vi "FPGA DAC IO Node.vi"(0 "data":T1[](array[typedef])=[{"I"=0.0, "Q"=0.0, "overflow"=FALSE}, {"I"=0.0, "Q"=0.0, "overflow"=FALSE}], 9 "input valid":bool, 11 "niUSRP Tx Core v1 FPGA.lvclass":refnum<class "niUSRP Tx Core v1 FPGA.lvclass">) -> ()   [LabVIEW 2025, in "niUSRP Tx Core v1 FPGA.lvclass"]
uses:
  niUSRP Tx Core v1 FPGA.lvclass
  <instrlib>/_niInstr/DSP/v1/Shared/Public/IQ Data.ctl
  <vilib>/rvi/eio/common/nirviEmuTemplateMethod_errors.vi
  <vilib>/eio/EIONode/EIONode.xnode
  <instrlib>/_niInstr/Basic Elements/v1/FPGA/niInstr Basic Elements v1 FPGA.lvlib
  <instrlib>/_niInstr/DSP/v1/Shared/niInstr DSP v1 Shared.lvlib
  <vilib>/rvi/DataTransferAndStorage/Container/XNode/niFpgaContainer.xnode
  <instrlib>/_niInstr/DSP/v1/FPGA/niInstr DSP v1 FPGA.lvlib
  <vilib>/rvi/FIFO/Fifo_Resource/niFpgaFifoEmulationRefIn.vi
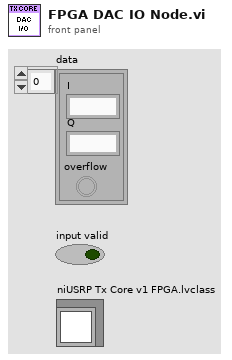
[diagram p1: front panel]
types:
  T1 = typedef "niInstr DSP v1 Shared.lvlib/IQ Data.ctl" = cluster{"I":fxp<+/-,18,1>, "Q":fxp<+/-,18,1>, "overflow":bool}
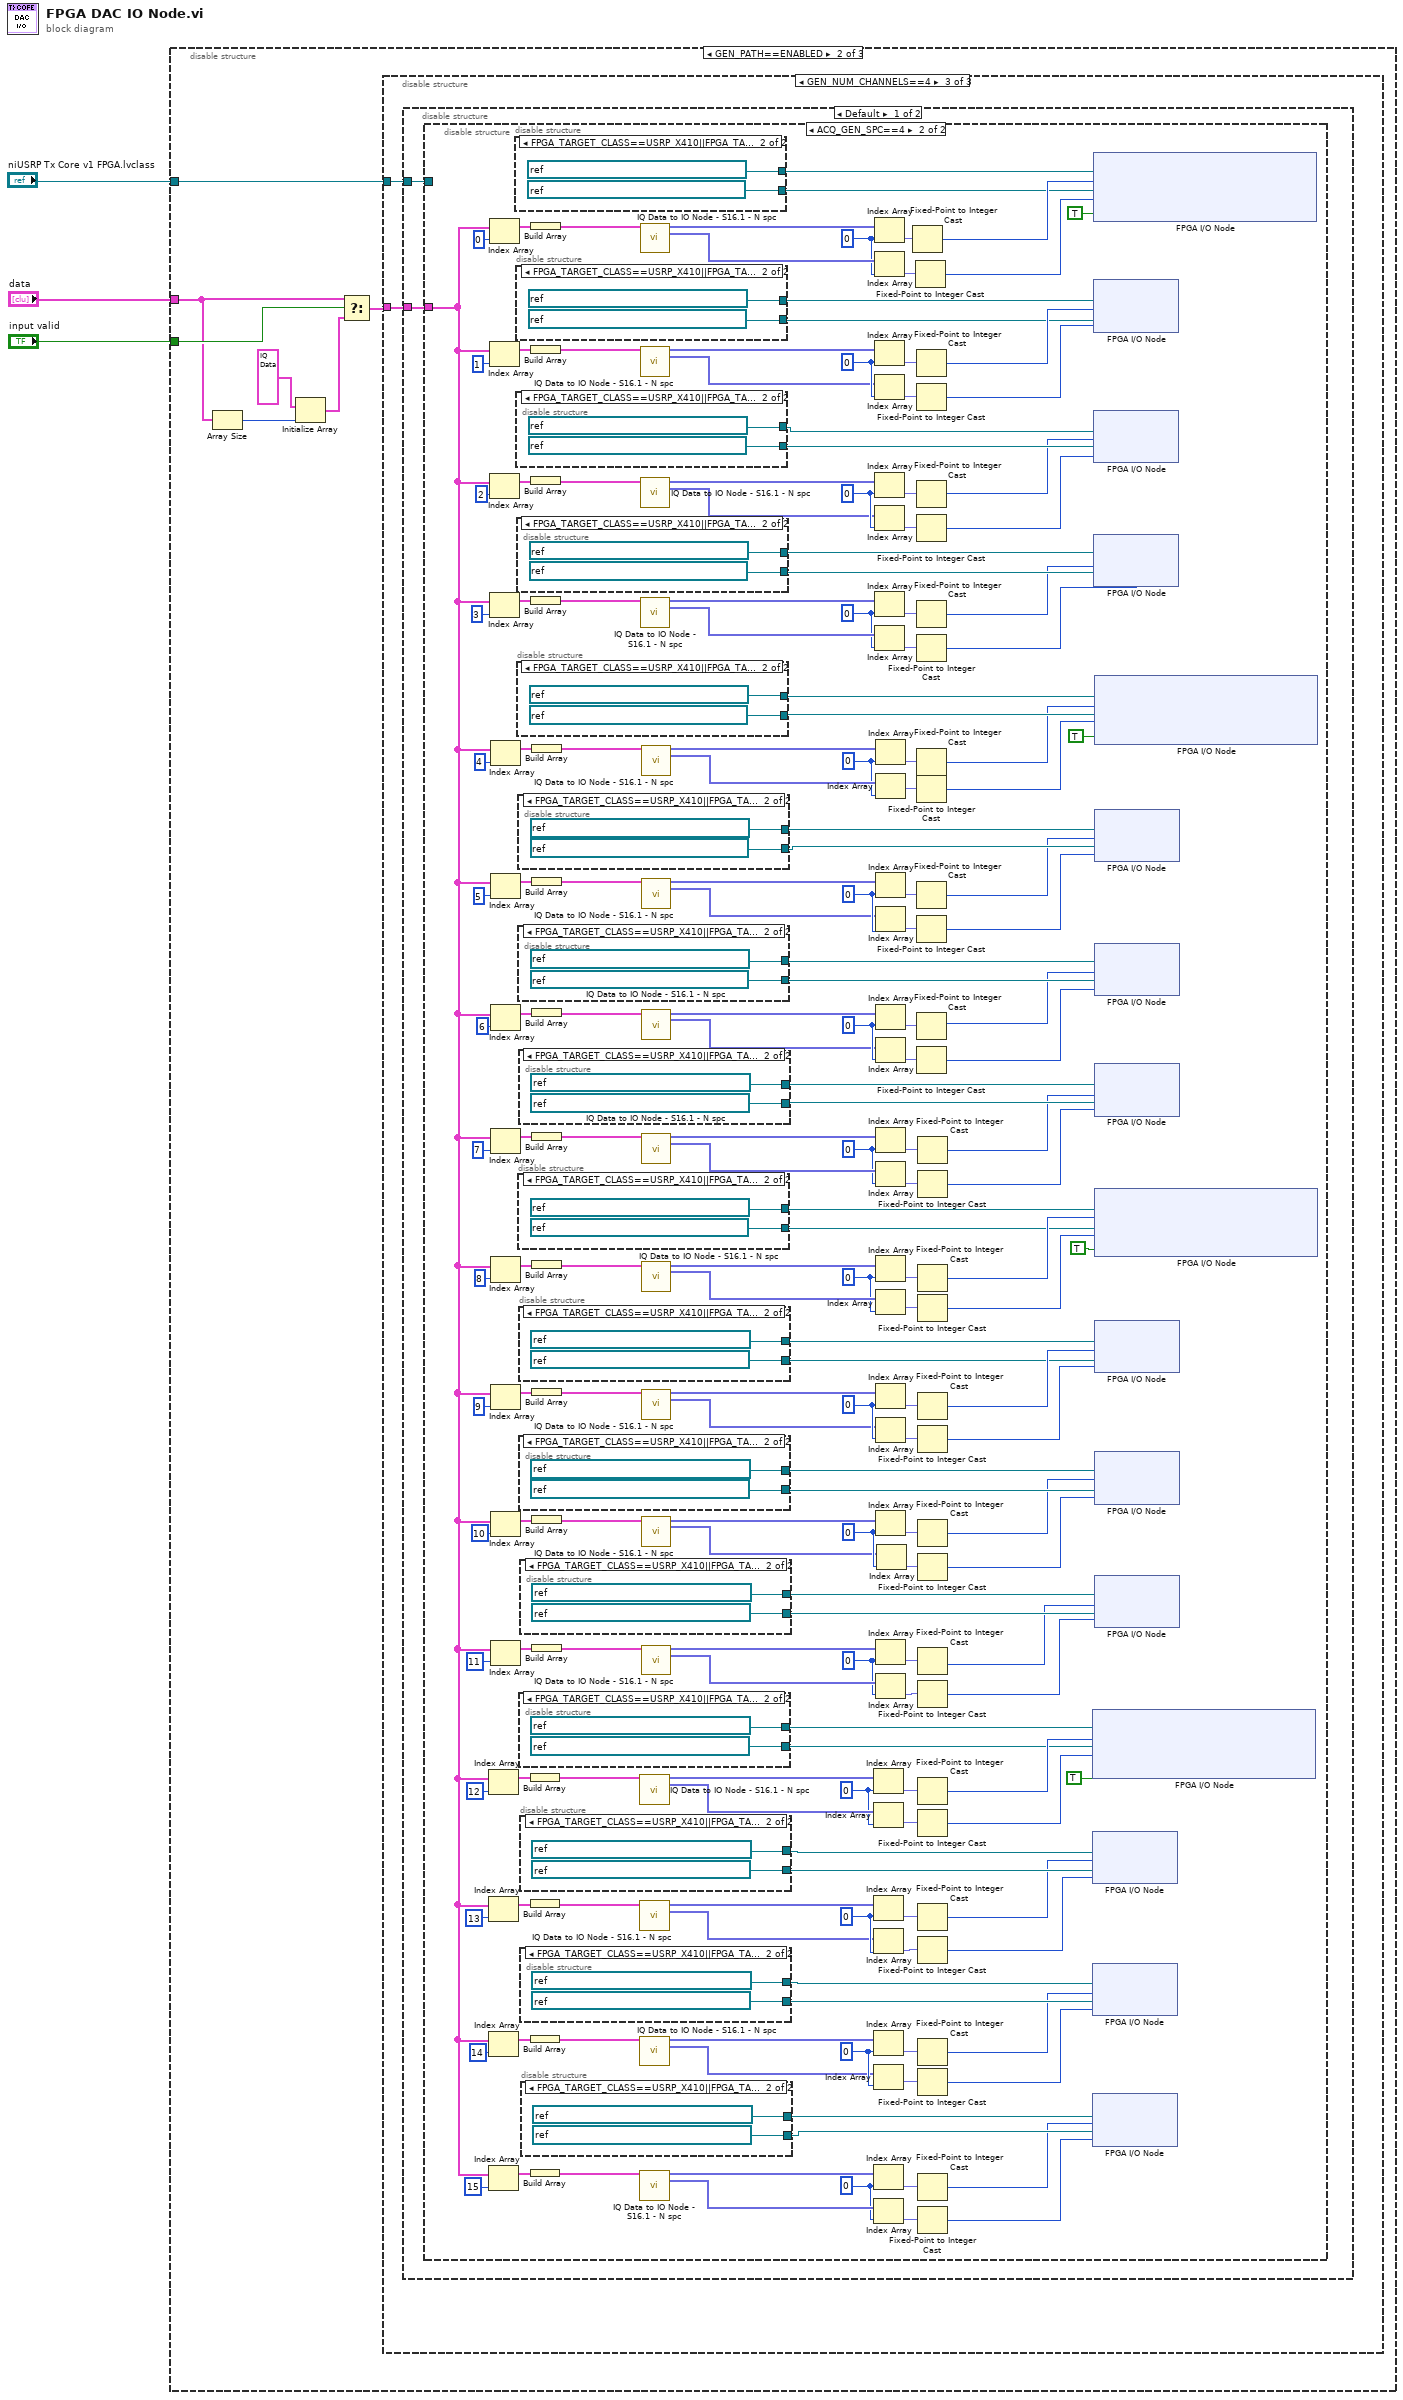
[diagram p0: block diagram]
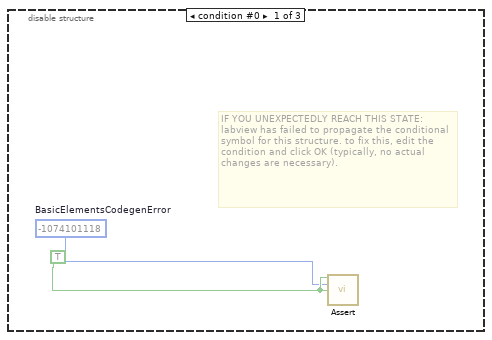
[diagram p2: hidden frame]
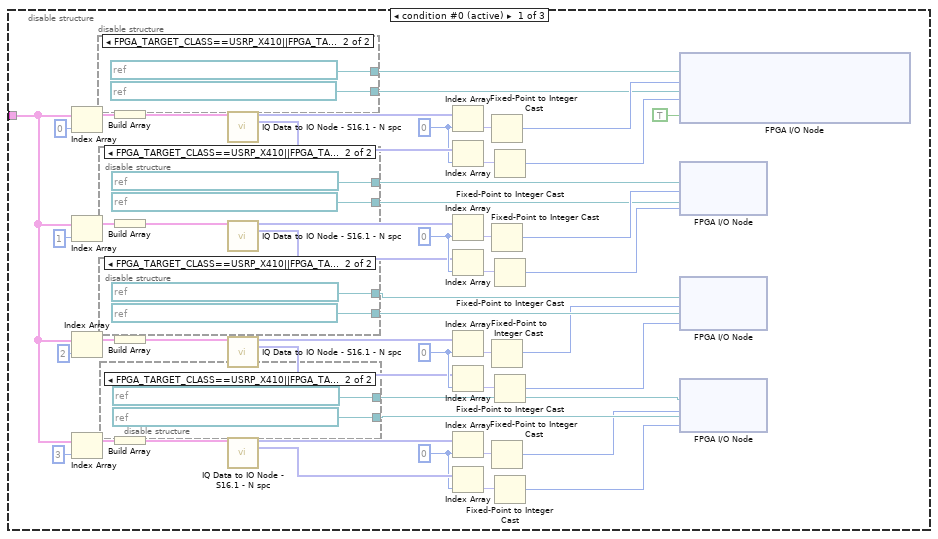
[diagram p4: hidden frame]
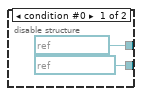
[diagram p5: hidden frame]
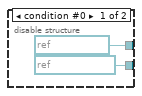
[diagram p6: hidden frame]
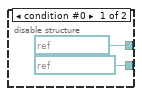
[diagram p7: hidden frame]
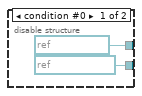
[diagram p8: hidden frame]
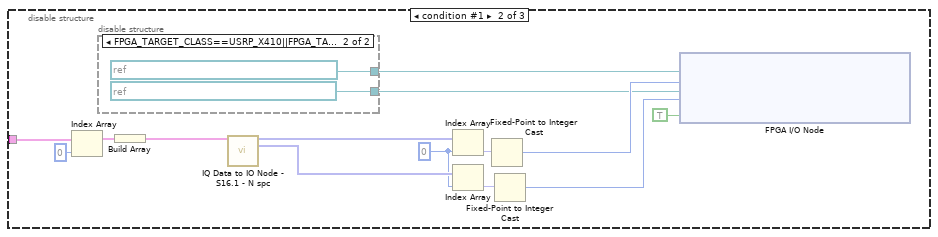
[diagram p9: hidden frame]
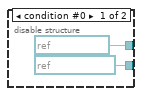
[diagram p10: hidden frame]
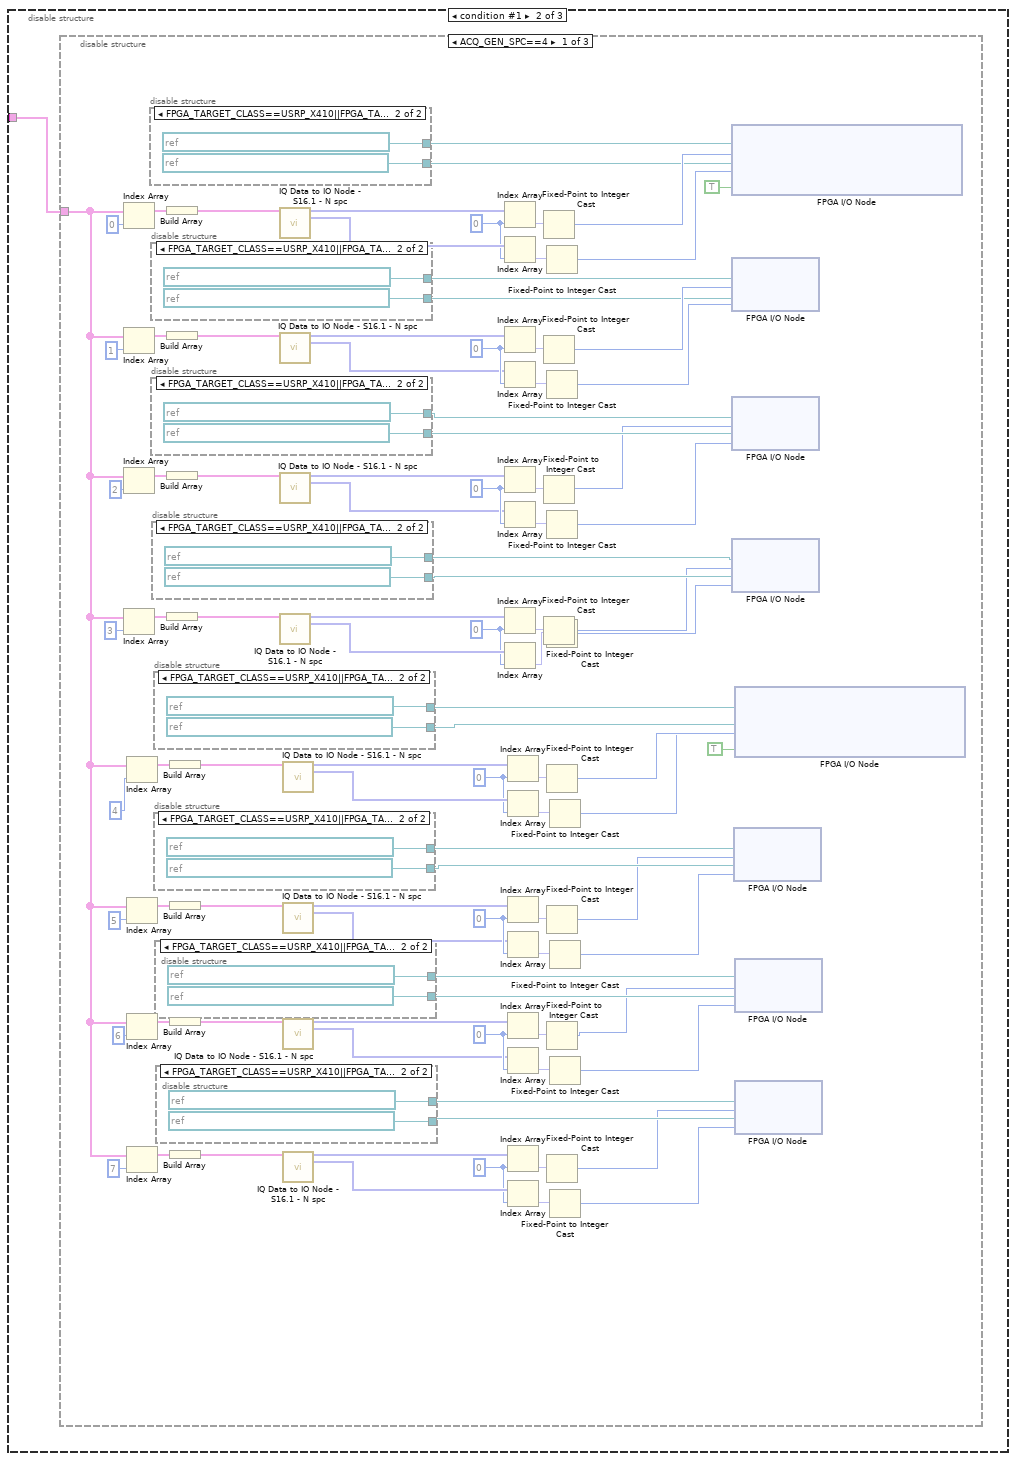
[diagram p11: hidden frame]
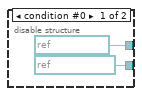
[diagram p12: hidden frame]
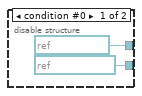
[diagram p13: hidden frame]
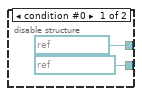
[diagram p14: hidden frame]
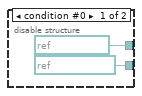
[diagram p15: hidden frame]
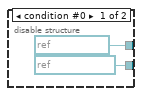
[diagram p16: hidden frame]
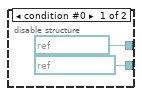
[diagram p17: hidden frame]
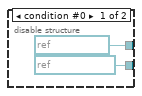
[diagram p18: hidden frame]
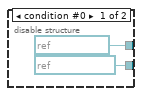
[diagram p19: hidden frame]
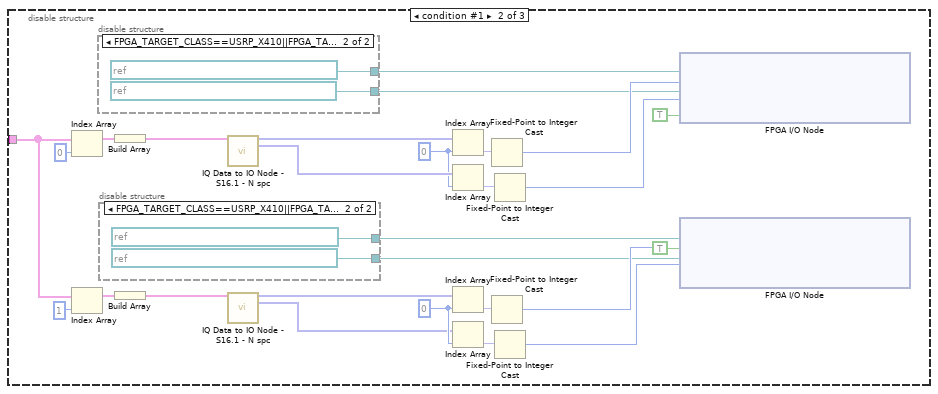
[diagram p20: hidden frame]
diagram:
  n1 = disable-structure shown="GEN_PATH==ENABLED" {
    disable-tunnel: "data" -> [_ w9 _]
    disable-tunnel: "input valid" -> [_ w11 _]
    disable-tunnel: "niUSRP Tx Core v1 FPGA.lvclass" -> [_ w12 _]
    frame condition #0 {
      w5 = TRUE ("assert")
      w4 = -1074101118  # BasicElementsCodegenError
      # "IF YOU UNEXPECTEDLY REACH THIS STATE:\nlabview has failed to propagate the conditional symbol for this structure. to fix this, edit the condition and click OK (typically, no actual changes are necessary)."
      n2 = call <instrlib>:"Assert.vi"("assert"=w5, "error code"=w4, "enable show error"=w5) -> ()  [unwired: 13 in]
    }
    frame condition #1 (active) {
      n3 = Array Size(array=w9) -> (size(s)=w7:i32)
      n4 = Initialize Array(T1 {"I"=0.0, "Q"=0.0, "overflow"=FALSE} ("data"), w7) -> (w6:T1[])
      n5 = Select(t=w9, s=w11, f=w6) -> (s? t:f=w10:T1[])
      n6 = disable-structure shown="GEN_NUM_CHANNELS==4" {
        disable-tunnel: w12 -> [_ _ w266]
        disable-tunnel: w10 -> [w13 w98 w265]
        frame condition #0 {
          n7 = disable-structure shown="Default" {
            disable-tunnel: w13 -> [w14 w80 _]
            frame condition #0 (active) {
              w39 = 0 ("index")
              w30 = 0 ("index")
              w49 = 0 ("index")
              w58 = 0 ("index")
              n8 = Index Array(array=w14, index=0) -> (element=w55:T1)
              n9 = Index Array(array=w14, index=1) -> (element=w50:T1)
              n10 = Index Array(array=w14, index=2) -> (element=w32:T1)
              n11 = Index Array(array=w14, index=3) -> (element=w37:T1)
              n12 = disable-structure shown="FPGA_TARGET_CLASS==USRP_X410||FPGA_TARGET_CLASS==USRP_X410__EMBEDDED____UNSUPPORTED" {
                disable-tunnel: [refnum<k21> "RF 0/Tx/I" ("tx regs.i out resource") refnum<k21> "Daughterboard 0\\RF 0.Tx.I0" ("FPGA I/O")] -> w25
                disable-tunnel: [refnum<k21> "RF 0/Tx/Q" ("tx regs.i out resource") refnum<k21> "Daughterboard 0\\RF 0.Tx.Q0" ("FPGA I/O")] -> w24
                frame condition #0 {
                }
                frame condition #1 (active) {
                }
              }
              n13 = disable-structure shown="FPGA_TARGET_CLASS==USRP_X410||FPGA_TARGET_CLASS==USRP_X410__EMBEDDED____UNSUPPORTED" {
                disable-tunnel: [refnum<k21> "RF 0/Tx/I" ("tx regs.i out resource") refnum<k21> "Daughterboard 0\\RF 0.Tx.I1" ("FPGA I/O")] -> w23
                disable-tunnel: [refnum<k21> "RF 0/Tx/Q" ("tx regs.i out resource") refnum<k21> "Daughterboard 0\\RF 0.Tx.Q1" ("FPGA I/O")] -> w22
                frame condition #0 {
                }
                frame condition #1 (active) {
                }
              }
              n14 = disable-structure shown="FPGA_TARGET_CLASS==USRP_X410||FPGA_TARGET_CLASS==USRP_X410__EMBEDDED____UNSUPPORTED" {
                disable-tunnel: [refnum<k21> "RF 0/Tx/I" ("tx regs.i out resource") refnum<k21> "Daughterboard 0\\RF 0.Tx.I2" ("FPGA I/O")] -> w21
                disable-tunnel: [refnum<k21> "RF 0/Tx/Q" ("tx regs.i out resource") refnum<k21> "Daughterboard 0\\RF 0.Tx.Q2" ("FPGA I/O")] -> w20
                frame condition #0 {
                }
                frame condition #1 (active) {
                }
              }
              n15 = disable-structure shown="FPGA_TARGET_CLASS==USRP_X410||FPGA_TARGET_CLASS==USRP_X410__EMBEDDED____UNSUPPORTED" {
                disable-tunnel: [refnum<k21> "RF 0/Tx/I" ("tx regs.i out resource") refnum<k21> "Daughterboard 0\\RF 0.Tx.I3" ("FPGA I/O")] -> w19
                disable-tunnel: [refnum<k21> "RF 0/Tx/Q" ("tx regs.i out resource") refnum<k21> "Daughterboard 0\\RF 0.Tx.Q3" ("FPGA I/O")] -> w18
                frame condition #0 {
                }
                frame condition #1 (active) {
                }
              }
              n16 = Build Array(w55) -> (w53:T1[])
              n17 = Build Array(w50) -> (w52:T1[])
              n18 = Build Array(w32) -> (w34:T1[])
              n19 = Build Array(w37) -> (w35:T1[])
              n20 = call "IQ Data to IO Node - S16.1 - N spc.vi"("data in"=w53) -> ("I out"=w63:fxp<+/-,16,1>[], "Q out"=w62:fxp<+/-,16,1>[])  [unwired: 12 in, 1 out]
              n21 = call "IQ Data to IO Node - S16.1 - N spc.vi"("data in"=w52) -> ("I out"=w44:fxp<+/-,16,1>[], "Q out"=w45:fxp<+/-,16,1>[])  [unwired: 12 in, 1 out]
              n22 = call "IQ Data to IO Node - S16.1 - N spc.vi"("data in"=w34) -> ("I out"=w26:fxp<+/-,16,1>[], "Q out"=w27:fxp<+/-,16,1>[])  [unwired: 12 in, 1 out]
              n23 = call "IQ Data to IO Node - S16.1 - N spc.vi"("data in"=w35) -> ("I out"=w43:fxp<+/-,16,1>[], "Q out"=w42:fxp<+/-,16,1>[])  [unwired: 12 in, 1 out]
              n24 = Index Array(array=w63, index=w58) -> (element=w61:fxp<+/-,16,1>)
              n25 = Index Array(array=w62, index=w58) -> (element=w59:fxp<+/-,16,1>)
              n26 = Index Array(array=w44, index=w49) -> (element=w46:fxp<+/-,16,1>)
              n27 = Index Array(array=w45, index=w49) -> (element=w48:fxp<+/-,16,1>)
              n28 = Index Array(array=w26, index=w30) -> (element=w28:fxp<+/-,16,1>)
              n29 = Index Array(array=w27, index=w30) -> (element=w29:fxp<+/-,16,1>)
              n30 = Index Array(array=w43, index=w39) -> (element=w41:fxp<+/-,16,1>)
              n31 = Index Array(array=w42, index=w39) -> (element=w40:fxp<+/-,16,1>)
              n32 = Fixed-Point to Integer Cast(1:w61) -> (0:w60:i16)
              n33 = Fixed-Point to Integer Cast(1:w46) -> (0:w47:i16)
              n34 = Fixed-Point to Integer Cast(1:w28) -> (0:w15:i16)
              n35 = Fixed-Point to Integer Cast(1:w41) -> (0:w17:i16)
              n36 = Fixed-Point to Integer Cast(1:w59) -> (0:w57:i16)
              n37 = Fixed-Point to Integer Cast(1:w48) -> (0:w16:i16)
              n38 = Fixed-Point to Integer Cast(1:w29) -> (0:w31:i16)
              n39 = Fixed-Point to Integer Cast(1:w40) -> (0:w38:i16)
              n40 = xnode "FPGA I/O Node"("I/O Item"=w60, "FPGA I/O In"=w25, "I/O Item"=w57, "FPGA I/O In"=w24, "Daughterboard 0\\RF 0.Tx.Data Valid"=TRUE ("Daughterboard 1\\s1TxDbaCh0DataValid")) -> ()  [unwired: 1 in, 3 out]
              n41 = xnode "FPGA I/O Node"("I/O Item"=w47, "FPGA I/O In"=w23, "I/O Item"=w16, "FPGA I/O In"=w22) -> ()  [unwired: 2 out]
              n42 = xnode "FPGA I/O Node"("I/O Item"=w15, "FPGA I/O In"=w21, "I/O Item"=w31, "FPGA I/O In"=w20) -> ()  [unwired: 2 out]
              n43 = xnode "FPGA I/O Node"("I/O Item"=w17, "FPGA I/O In"=w19, "I/O Item"=w38, "FPGA I/O In"=w18) -> ()  [unwired: 2 out]
            }
            frame condition #1 {
              w88 = 0 ("index")
              n44 = Index Array(array=w80, index=0) -> (element=w85:T1)
              n45 = disable-structure shown="FPGA_TARGET_CLASS==USRP_X410||FPGA_TARGET_CLASS==USRP_X410__EMBEDDED____UNSUPPORTED" {
                disable-tunnel: [refnum<k21> "RF 0/Tx/I" ("tx regs.i out resource") refnum<k21> "Daughterboard 0\\RF 0.Tx.I" ("FPGA I/O")] -> w82
                disable-tunnel: [refnum<k21> "RF 0/Tx/Q" ("tx regs.i out resource") refnum<k21> "Daughterboard 0\\RF 0.Tx.Q" ("FPGA I/O")] -> w81
                frame condition #0 {
                }
                frame condition #1 (active) {
                }
              }
              n46 = Build Array(w85) -> (w83:T1[])
              n47 = call "IQ Data to IO Node - S16.1 - N spc.vi"("data in"=w83) -> ("I out"=w93:fxp<+/-,16,1>[], "Q out"=w92:fxp<+/-,16,1>[])  [unwired: 12 in, 1 out]
              n48 = Index Array(array=w93, index=w88) -> (element=w91:fxp<+/-,16,1>)
              n49 = Index Array(array=w92, index=w88) -> (element=w89:fxp<+/-,16,1>)
              n50 = Fixed-Point to Integer Cast(1:w91) -> (0:w90:i16)
              n51 = Fixed-Point to Integer Cast(1:w89) -> (0:w87:i16)
              n52 = xnode "FPGA I/O Node"("I/O Item"=w90, "FPGA I/O In"=w82, "I/O Item"=w87, "FPGA I/O In"=w81, "Daughterboard 0\\RF 0.Tx.Data Valid"=TRUE ("Daughterboard 1\\s1TxDbaCh0DataValid")) -> ()  [unwired: 1 in, 3 out]
            }
            frame condition #2 {
            }
          }
        }
        frame condition #1 {
          n53 = disable-structure shown="ACQ_GEN_SPC==4" {
            disable-tunnel: w98 -> [w101 w230 _]
            frame condition #0 (active) {
              w127 = 0 ("index")
              w119 = 0 ("index")
              w135 = 0 ("index")
              w144 = 0 ("index")
              w173 = 0 ("index")
              w164 = 0 ("index")
              w183 = 0 ("index")
              w192 = 0 ("index")
              n54 = Index Array(array=w101, index=0) -> (element=w189:T1)
              n55 = Index Array(array=w101, index=1) -> (element=w184:T1)
              n56 = Index Array(array=w101, index=2) -> (element=w166:T1)
              n57 = Index Array(array=w101, index=3) -> (element=w171:T1)
              n58 = Index Array(array=w101, index=4) -> (element=w142:T1)
              n59 = Index Array(array=w101, index=5) -> (element=w137:T1)
              n60 = Index Array(array=w101, index=6) -> (element=w121:T1)
              n61 = Index Array(array=w101, index=7) -> (element=w126:T1)
              n62 = disable-structure shown="FPGA_TARGET_CLASS==USRP_X410||FPGA_TARGET_CLASS==USRP_X410__EMBEDDED____UNSUPPORTED" {
                disable-tunnel: [refnum<k21> "RF 0/Tx/I" ("tx regs.i out resource") refnum<k21> "Daughterboard 0\\RF 0.Tx.I0" ("FPGA I/O")] -> w159
                disable-tunnel: [refnum<k21> "RF 0/Tx/Q" ("tx regs.i out resource") refnum<k21> "Daughterboard 0\\RF 0.Tx.Q0" ("FPGA I/O")] -> w158
                frame condition #0 {
                }
                frame condition #1 (active) {
                }
              }
              n63 = disable-structure shown="FPGA_TARGET_CLASS==USRP_X410||FPGA_TARGET_CLASS==USRP_X410__EMBEDDED____UNSUPPORTED" {
                disable-tunnel: [refnum<k21> "RF 0/Tx/I" ("tx regs.i out resource") refnum<k21> "Daughterboard 0\\RF 0.Tx.I1" ("FPGA I/O")] -> w157
                disable-tunnel: [refnum<k21> "RF 0/Tx/Q" ("tx regs.i out resource") refnum<k21> "Daughterboard 0\\RF 0.Tx.Q1" ("FPGA I/O")] -> w156
                frame condition #0 {
                }
                frame condition #1 (active) {
                }
              }
              n64 = disable-structure shown="FPGA_TARGET_CLASS==USRP_X410||FPGA_TARGET_CLASS==USRP_X410__EMBEDDED____UNSUPPORTED" {
                disable-tunnel: [refnum<k21> "RF 0/Tx/I" ("tx regs.i out resource") refnum<k21> "Daughterboard 0\\RF 0.Tx.I2" ("FPGA I/O")] -> w155
                disable-tunnel: [refnum<k21> "RF 0/Tx/Q" ("tx regs.i out resource") refnum<k21> "Daughterboard 0\\RF 0.Tx.Q2" ("FPGA I/O")] -> w154
                frame condition #0 {
                }
                frame condition #1 (active) {
                }
              }
              n65 = disable-structure shown="FPGA_TARGET_CLASS==USRP_X410||FPGA_TARGET_CLASS==USRP_X410__EMBEDDED____UNSUPPORTED" {
                disable-tunnel: [refnum<k21> "RF 0/Tx/I" ("tx regs.i out resource") refnum<k21> "Daughterboard 0\\RF 0.Tx.I3" ("FPGA I/O")] -> w153
                disable-tunnel: [refnum<k21> "RF 0/Tx/Q" ("tx regs.i out resource") refnum<k21> "Daughterboard 0\\RF 0.Tx.Q3" ("FPGA I/O")] -> w152
                frame condition #0 {
                }
                frame condition #1 (active) {
                }
              }
              n66 = disable-structure shown="FPGA_TARGET_CLASS==USRP_X410||FPGA_TARGET_CLASS==USRP_X410__EMBEDDED____UNSUPPORTED" {
                disable-tunnel: [refnum<k21> "RF 0/Tx/I" ("tx regs.i out resource") refnum<k21> "Daughterboard 0\\RF 1.Tx.I0" ("FPGA I/O")] -> w114
                disable-tunnel: [refnum<k21> "RF 0/Tx/Q" ("tx regs.i out resource") refnum<k21> "Daughterboard 0\\RF 1.Tx.Q0" ("FPGA I/O")] -> w113
                frame condition #0 {
                }
                frame condition #1 (active) {
                }
              }
              n67 = disable-structure shown="FPGA_TARGET_CLASS==USRP_X410||FPGA_TARGET_CLASS==USRP_X410__EMBEDDED____UNSUPPORTED" {
                disable-tunnel: [refnum<k21> "RF 0/Tx/I" ("tx regs.i out resource") refnum<k21> "Daughterboard 0\\RF 1.Tx.I1" ("FPGA I/O")] -> w112
                disable-tunnel: [refnum<k21> "RF 0/Tx/Q" ("tx regs.i out resource") refnum<k21> "Daughterboard 0\\RF 1.Tx.Q1" ("FPGA I/O")] -> w111
                frame condition #0 {
                }
                frame condition #1 (active) {
                }
              }
              n68 = disable-structure shown="FPGA_TARGET_CLASS==USRP_X410||FPGA_TARGET_CLASS==USRP_X410__EMBEDDED____UNSUPPORTED" {
                disable-tunnel: [refnum<k21> "RF 0/Tx/I" ("tx regs.i out resource") refnum<k21> "Daughterboard 0\\RF 1.Tx.I2" ("FPGA I/O")] -> w110
                disable-tunnel: [refnum<k21> "RF 0/Tx/Q" ("tx regs.i out resource") refnum<k21> "Daughterboard 0\\RF 1.Tx.Q2" ("FPGA I/O")] -> w109
                frame condition #0 {
                }
                frame condition #1 (active) {
                }
              }
              n69 = disable-structure shown="FPGA_TARGET_CLASS==USRP_X410||FPGA_TARGET_CLASS==USRP_X410__EMBEDDED____UNSUPPORTED" {
                disable-tunnel: [refnum<k21> "RF 0/Tx/I" ("tx regs.i out resource") refnum<k21> "Daughterboard 0\\RF 1.Tx.I3" ("FPGA I/O")] -> w108
                disable-tunnel: [refnum<k21> "RF 0/Tx/Q" ("tx regs.i out resource") refnum<k21> "Daughterboard 0\\RF 1.Tx.Q3" ("FPGA I/O")] -> w107
                frame condition #0 {
                }
                frame condition #1 (active) {
                }
              }
              n70 = Build Array(w189) -> (w187:T1[])
              n71 = Build Array(w184) -> (w186:T1[])
              n72 = Build Array(w166) -> (w168:T1[])
              n73 = Build Array(w171) -> (w169:T1[])
              n74 = Build Array(w142) -> (w140:T1[])
              n75 = Build Array(w137) -> (w139:T1[])
              n76 = Build Array(w121) -> (w123:T1[])
              n77 = Build Array(w126) -> (w124:T1[])
              n78 = call "IQ Data to IO Node - S16.1 - N spc.vi"("data in"=w187) -> ("I out"=w197:fxp<+/-,16,1>[], "Q out"=w196:fxp<+/-,16,1>[])  [unwired: 12 in, 1 out]
              n79 = call "IQ Data to IO Node - S16.1 - N spc.vi"("data in"=w186) -> ("I out"=w178:fxp<+/-,16,1>[], "Q out"=w179:fxp<+/-,16,1>[])  [unwired: 12 in, 1 out]
              n80 = call "IQ Data to IO Node - S16.1 - N spc.vi"("data in"=w168) -> ("I out"=w160:fxp<+/-,16,1>[], "Q out"=w161:fxp<+/-,16,1>[])  [unwired: 12 in, 1 out]
              n81 = call "IQ Data to IO Node - S16.1 - N spc.vi"("data in"=w169) -> ("I out"=w177:fxp<+/-,16,1>[], "Q out"=w176:fxp<+/-,16,1>[])  [unwired: 12 in, 1 out]
              n82 = call "IQ Data to IO Node - S16.1 - N spc.vi"("data in"=w140) -> ("I out"=w148:fxp<+/-,16,1>[], "Q out"=w147:fxp<+/-,16,1>[])  [unwired: 12 in, 1 out]
              n83 = call "IQ Data to IO Node - S16.1 - N spc.vi"("data in"=w139) -> ("I out"=w131:fxp<+/-,16,1>[], "Q out"=w132:fxp<+/-,16,1>[])  [unwired: 12 in, 1 out]
              n84 = call "IQ Data to IO Node - S16.1 - N spc.vi"("data in"=w123) -> ("I out"=w115:fxp<+/-,16,1>[], "Q out"=w116:fxp<+/-,16,1>[])  [unwired: 12 in, 1 out]
              n85 = call "IQ Data to IO Node - S16.1 - N spc.vi"("data in"=w124) -> ("I out"=w130:fxp<+/-,16,1>[], "Q out"=w129:fxp<+/-,16,1>[])  [unwired: 12 in, 1 out]
              n86 = Index Array(array=w197, index=w192) -> (element=w195:fxp<+/-,16,1>)
              n87 = Index Array(array=w196, index=w192) -> (element=w193:fxp<+/-,16,1>)
              n88 = Index Array(array=w178, index=w183) -> (element=w180:fxp<+/-,16,1>)
              n89 = Index Array(array=w179, index=w183) -> (element=w182:fxp<+/-,16,1>)
              n90 = Index Array(array=w160, index=w164) -> (element=w162:fxp<+/-,16,1>)
              n91 = Index Array(array=w161, index=w164) -> (element=w163:fxp<+/-,16,1>)
              n92 = Index Array(array=w177, index=w173) -> (element=w175:fxp<+/-,16,1>)
              n93 = Index Array(array=w176, index=w173) -> (element=w174:fxp<+/-,16,1>)
              n94 = Index Array(array=w148, index=w144) -> (element=w146:fxp<+/-,16,1>)
              n95 = Index Array(array=w147, index=w144) -> (element=w145:fxp<+/-,16,1>)
              n96 = Index Array(array=w131, index=w135) -> (element=w133:fxp<+/-,16,1>)
              n97 = Index Array(array=w132, index=w135) -> (element=w134:fxp<+/-,16,1>)
              n98 = Index Array(array=w115, index=w119) -> (element=w117:fxp<+/-,16,1>)
              n99 = Index Array(array=w116, index=w119) -> (element=w118:fxp<+/-,16,1>)
              n100 = Index Array(array=w130, index=w127) -> (element=w128:fxp<+/-,16,1>)
              n101 = Index Array(array=w129, index=w127) -> (element=w100:fxp<+/-,16,1>)
              n102 = Fixed-Point to Integer Cast(1:w195) -> (0:w194:i16)
              n103 = Fixed-Point to Integer Cast(1:w180) -> (0:w181:i16)
              n104 = Fixed-Point to Integer Cast(1:w162) -> (0:w149:i16)
              n105 = Fixed-Point to Integer Cast(1:w175) -> (0:w151:i16)
              n106 = Fixed-Point to Integer Cast(1:w193) -> (0:w191:i16)
              n107 = Fixed-Point to Integer Cast(1:w182) -> (0:w150:i16)
              n108 = Fixed-Point to Integer Cast(1:w163) -> (0:w165:i16)
              n109 = Fixed-Point to Integer Cast(1:w174) -> (0:w172:i16)
              n110 = Fixed-Point to Integer Cast(1:w146) -> (0:w105:i16)
              n111 = Fixed-Point to Integer Cast(1:w133) -> (0:w103:i16)
              n112 = Fixed-Point to Integer Cast(1:w117) -> (0:w102:i16)
              n113 = Fixed-Point to Integer Cast(1:w128) -> (0:w106:i16)
              n114 = Fixed-Point to Integer Cast(1:w145) -> (0:w104:i16)
              n115 = Fixed-Point to Integer Cast(1:w134) -> (0:w136:i16)
              n116 = Fixed-Point to Integer Cast(1:w118) -> (0:w120:i16)
              n117 = Fixed-Point to Integer Cast(1:w100) -> (0:w99:i16)
              n118 = xnode "FPGA I/O Node"("I/O Item"=w194, "FPGA I/O In"=w159, "I/O Item"=w191, "FPGA I/O In"=w158, "Daughterboard 0\\RF 0.Tx.Data Valid"=TRUE ("Daughterboard 1\\s1TxDbaCh0DataValid")) -> ()  [unwired: 1 in, 3 out]
              n119 = xnode "FPGA I/O Node"("I/O Item"=w181, "FPGA I/O In"=w157, "I/O Item"=w150, "FPGA I/O In"=w156) -> ()  [unwired: 2 out]
              n120 = xnode "FPGA I/O Node"("I/O Item"=w149, "FPGA I/O In"=w155, "I/O Item"=w165, "FPGA I/O In"=w154) -> ()  [unwired: 2 out]
              n121 = xnode "FPGA I/O Node"("I/O Item"=w151, "FPGA I/O In"=w153, "I/O Item"=w172, "FPGA I/O In"=w152) -> ()  [unwired: 2 out]
              n122 = xnode "FPGA I/O Node"("I/O Item"=w103, "FPGA I/O In"=w112, "I/O Item"=w136, "FPGA I/O In"=w111) -> ()  [unwired: 2 out]
              n123 = xnode "FPGA I/O Node"("I/O Item"=w105, "FPGA I/O In"=w114, "I/O Item"=w104, "FPGA I/O In"=w113, "Daughterboard 0\\RF 1.Tx.Data Valid"=TRUE ("Daughterboard 1\\s1TxDbaCh0DataValid")) -> ()  [unwired: 1 in, 3 out]
              n124 = xnode "FPGA I/O Node"("I/O Item"=w102, "FPGA I/O In"=w110, "I/O Item"=w120, "FPGA I/O In"=w109) -> ()  [unwired: 2 out]
              n125 = xnode "FPGA I/O Node"("I/O Item"=w106, "FPGA I/O In"=w108, "I/O Item"=w99, "FPGA I/O In"=w107) -> ()  [unwired: 2 out]
            }
            frame condition #1 {
              w241 = 0 ("index")
              w251 = 0 ("index")
              n126 = Index Array(array=w230, index=0) -> (element=w248:T1)
              n127 = Index Array(array=w230, index=1) -> (element=w243:T1)
              n128 = disable-structure shown="FPGA_TARGET_CLASS==USRP_X410||FPGA_TARGET_CLASS==USRP_X410__EMBEDDED____UNSUPPORTED" {
                disable-tunnel: [refnum<k21> "RF 0/Tx/I" ("tx regs.i out resource") refnum<k21> "Daughterboard 0\\RF 0.Tx.I" ("FPGA I/O")] -> w235
                disable-tunnel: [refnum<k21> "RF 0/Tx/Q" ("tx regs.i out resource") refnum<k21> "Daughterboard 0\\RF 0.Tx.Q" ("FPGA I/O")] -> w234
                frame condition #0 {
                }
                frame condition #1 (active) {
                }
              }
              n129 = disable-structure shown="FPGA_TARGET_CLASS==USRP_X410||FPGA_TARGET_CLASS==USRP_X410__EMBEDDED____UNSUPPORTED" {
                disable-tunnel: [refnum<k21> "RF 0/Tx/I" ("tx regs.i out resource") refnum<k21> "Daughterboard 0\\RF 1.Tx.I" ("FPGA I/O")] -> w233
                disable-tunnel: [refnum<k21> "RF 0/Tx/Q" ("tx regs.i out resource") refnum<k21> "Daughterboard 0\\RF 1.Tx.Q" ("FPGA I/O")] -> w232
                frame condition #0 {
                }
                frame condition #1 (active) {
                }
              }
              n130 = Build Array(w248) -> (w246:T1[])
              n131 = Build Array(w243) -> (w245:T1[])
              n132 = call "IQ Data to IO Node - S16.1 - N spc.vi"("data in"=w246) -> ("I out"=w256:fxp<+/-,16,1>[], "Q out"=w255:fxp<+/-,16,1>[])  [unwired: 12 in, 1 out]
              n133 = call "IQ Data to IO Node - S16.1 - N spc.vi"("data in"=w245) -> ("I out"=w236:fxp<+/-,16,1>[], "Q out"=w237:fxp<+/-,16,1>[])  [unwired: 12 in, 1 out]
              n134 = Index Array(array=w256, index=w251) -> (element=w254:fxp<+/-,16,1>)
              n135 = Index Array(array=w255, index=w251) -> (element=w252:fxp<+/-,16,1>)
              n136 = Index Array(array=w236, index=w241) -> (element=w238:fxp<+/-,16,1>)
              n137 = Index Array(array=w237, index=w241) -> (element=w240:fxp<+/-,16,1>)
              n138 = Fixed-Point to Integer Cast(1:w254) -> (0:w253:i16)
              n139 = Fixed-Point to Integer Cast(1:w238) -> (0:w239:i16)
              n140 = Fixed-Point to Integer Cast(1:w252) -> (0:w250:i16)
              n141 = Fixed-Point to Integer Cast(1:w240) -> (0:w231:i16)
              n142 = xnode "FPGA I/O Node"("I/O Item"=w253, "FPGA I/O In"=w235, "I/O Item"=w250, "FPGA I/O In"=w234, "Daughterboard 0\\RF 0.Tx.Data Valid"=TRUE ("Daughterboard 1\\s1TxDbaCh0DataValid")) -> ()  [unwired: 1 in, 3 out]
              n143 = xnode "FPGA I/O Node"("I/O Item"=w239, "FPGA I/O In"=w233, "I/O Item"=w231, "FPGA I/O In"=w232, "Daughterboard 0\\RF 1.Tx.Data Valid"=TRUE ("Daughterboard 1\\s1TxDbaCh0DataValid")) -> ()  [unwired: 1 in, 3 out]
            }
            frame condition #2 {
            }
          }
        }
        frame condition #2 (active) {
          n144 = disable-structure shown="Default" {
            disable-tunnel: w266 -> [w268 w612]
            disable-tunnel: w265 -> [w267 w611]
            frame condition #0 (active) {
              n145 = disable-structure shown="ACQ_GEN_SPC==4" {
                disable-tunnel: w268 -> [_ _]
                disable-tunnel: w267 -> [w269 w389]
                frame condition #0 {
                  w296 = 0 ("index")
                  w285 = 0 ("index")
                  w306 = 0 ("index")
                  w316 = 0 ("index")
                  n146 = Index Array(array=w269, index=0) -> (element=w313:T1)
                  n147 = Index Array(array=w269, index=1) -> (element=w308:T1)
                  n148 = Index Array(array=w269, index=2) -> (element=w288:T1)
                  n149 = Index Array(array=w269, index=3) -> (element=w293:T1)
                  n150 = disable-structure shown="FPGA_TARGET_CLASS==USRP_X410||FPGA_TARGET_CLASS==USRP_X410__EMBEDDED____UNSUPPORTED" {
                    disable-tunnel: [refnum<k21> "RF 0/Tx/I" ("tx regs.i out resource") refnum<k21> "Daughterboard 0\\RF 0.Tx.I" ("FPGA I/O")] -> w280
                    disable-tunnel: [refnum<k21> "RF 0/Tx/Q" ("tx regs.i out resource") refnum<k21> "Daughterboard 0\\RF 0.Tx.Q" ("FPGA I/O")] -> w279
                    frame condition #0 {
                    }
                    frame condition #1 (active) {
                    }
                  }
                  n151 = disable-structure shown="FPGA_TARGET_CLASS==USRP_X410||FPGA_TARGET_CLASS==USRP_X410__EMBEDDED____UNSUPPORTED" {
                    disable-tunnel: [refnum<k21> "RF 0/Tx/I" ("tx regs.i out resource") refnum<k21> "Daughterboard 0\\RF 1.Tx.I" ("FPGA I/O")] -> w278
                    disable-tunnel: [refnum<k21> "RF 0/Tx/Q" ("tx regs.i out resource") refnum<k21> "Daughterboard 0\\RF 1.Tx.Q" ("FPGA I/O")] -> w277
                    frame condition #0 {
                    }
                    frame condition #1 (active) {
                    }
                  }
                  n152 = disable-structure shown="FPGA_TARGET_CLASS==USRP_X410||FPGA_TARGET_CLASS==USRP_X410__EMBEDDED____UNSUPPORTED" {
                    disable-tunnel: [refnum<k21> "RF 0/Tx/I" ("tx regs.i out resource") refnum<k21> "Daughterboard 1\\RF 0.Tx.I" ("FPGA I/O")] -> w276
                    disable-tunnel: [refnum<k21> "RF 0/Tx/Q" ("tx regs.i out resource") refnum<k21> "Daughterboard 1\\RF 0.Tx.Q" ("FPGA I/O")] -> w275
                    frame condition #0 {
                    }
                    frame condition #1 (active) {
                    }
                  }
                  n153 = disable-structure shown="FPGA_TARGET_CLASS==USRP_X410||FPGA_TARGET_CLASS==USRP_X410__EMBEDDED____UNSUPPORTED" {
                    disable-tunnel: [refnum<k21> "RF 0/Tx/I" ("tx regs.i out resource") refnum<k21> "Daughterboard 1\\RF 1.Tx.I" ("FPGA I/O")] -> w274
                    disable-tunnel: [refnum<k21> "RF 0/Tx/Q" ("tx regs.i out resource") refnum<k21> "Daughterboard 1\\RF 1.Tx.Q" ("FPGA I/O")] -> w273
                    frame condition #0 {
                    }
                    frame condition #1 (active) {
                    }
                  }
                  n154 = Build Array(w308) -> (w310:T1[])
                  n155 = Build Array(w288) -> (w290:T1[])
                  n156 = Build Array(w293) -> (w291:T1[])
                  n157 = Build Array(w313) -> (w311:T1[])
                  n158 = call "IQ Data to IO Node - S16.1 - N spc.vi"("data in"=w311) -> ("I out"=w321:fxp<+/-,16,1>[], "Q out"=w320:fxp<+/-,16,1>[])  [unwired: 12 in, 1 out]
                  n159 = call "IQ Data to IO Node - S16.1 - N spc.vi"("data in"=w310) -> ("I out"=w301:fxp<+/-,16,1>[], "Q out"=w302:fxp<+/-,16,1>[])  [unwired: 12 in, 1 out]
                  n160 = call "IQ Data to IO Node - S16.1 - N spc.vi"("data in"=w290) -> ("I out"=w281:fxp<+/-,16,1>[], "Q out"=w282:fxp<+/-,16,1>[])  [unwired: 12 in, 1 out]
                  n161 = call "IQ Data to IO Node - S16.1 - N spc.vi"("data in"=w291) -> ("I out"=w300:fxp<+/-,16,1>[], "Q out"=w299:fxp<+/-,16,1>[])  [unwired: 12 in, 1 out]
                  n162 = Index Array(array=w321, index=w316) -> (element=w319:fxp<+/-,16,1>)
                  n163 = Index Array(array=w320, index=w316) -> (element=w317:fxp<+/-,16,1>)
                  n164 = Index Array(array=w301, index=w306) -> (element=w303:fxp<+/-,16,1>)
                  n165 = Index Array(array=w302, index=w306) -> (element=w305:fxp<+/-,16,1>)
                  n166 = Index Array(array=w281, index=w285) -> (element=w283:fxp<+/-,16,1>)
                  n167 = Index Array(array=w282, index=w285) -> (element=w284:fxp<+/-,16,1>)
                  n168 = Index Array(array=w300, index=w296) -> (element=w298:fxp<+/-,16,1>)
                  n169 = Index Array(array=w299, index=w296) -> (element=w297:fxp<+/-,16,1>)
                  n170 = Fixed-Point to Integer Cast(1:w319) -> (0:w318:i16)
                  n171 = Fixed-Point to Integer Cast(1:w303) -> (0:w304:i16)
                  n172 = Fixed-Point to Integer Cast(1:w283) -> (0:w270:i16)
                  n173 = Fixed-Point to Integer Cast(1:w298) -> (0:w272:i16)
                  n174 = Fixed-Point to Integer Cast(1:w317) -> (0:w315:i16)
                  n175 = Fixed-Point to Integer Cast(1:w305) -> (0:w271:i16)
                  n176 = Fixed-Point to Integer Cast(1:w284) -> (0:w286:i16)
                  n177 = Fixed-Point to Integer Cast(1:w297) -> (0:w295:i16)
                  n178 = xnode "FPGA I/O Node"("I/O Item"=w318, "FPGA I/O In"=w280, "I/O Item"=w315, "FPGA I/O In"=w279, "Daughterboard 0\\RF 0.Tx.Data Valid"=TRUE ("Daughterboard 1\\s1TxDbaCh0DataValid")) -> ()  [unwired: 1 in, 3 out]
                  n179 = xnode "FPGA I/O Node"("I/O Item"=w304, "FPGA I/O In"=w278, "I/O Item"=w271, "FPGA I/O In"=w277, "Daughterboard 0\\RF 1.Tx.Data Valid"=TRUE ("Daughterboard 1\\s1TxDbaCh0DataValid")) -> ()  [unwired: 1 in, 3 out]
                  n180 = xnode "FPGA I/O Node"("I/O Item"=w270, "FPGA I/O In"=w276, "I/O Item"=w286, "FPGA I/O In"=w275, "Daughterboard 1\\RF 0.Tx.Data Valid"=TRUE ("Daughterboard 1\\s1TxDbaCh0DataValid")) -> ()  [unwired: 1 in, 3 out]
                  n181 = xnode "FPGA I/O Node"("I/O Item"=w272, "FPGA I/O In"=w274, "I/O Item"=w295, "FPGA I/O In"=w273, "Daughterboard 1\\RF 1.Tx.Data Valid"=TRUE ("Daughterboard 1\\s1TxDbaCh0DataValid")) -> ()  [unwired: 1 in, 3 out]
                }
                frame condition #1 (active) {
                  w401 = 0 ("index")
                  w394 = 0 ("index")
                  w410 = 0 ("index")
                  w419 = 0 ("index")
                  w436 = 0 ("index")
                  w429 = 0 ("index")
                  w446 = 0 ("index")
                  w455 = 0 ("index")
                  w474 = 0 ("index")
                  w465 = 0 ("index")
                  w483 = 0 ("index")
                  w492 = 0 ("index")
                  w510 = 0 ("index")
                  w501 = 0 ("index")
                  w520 = 0 ("index")
                  w529 = 0 ("index")
                  n182 = Index Array(array=w389, index=12) -> (element=w416:T1)
                  n183 = Index Array(array=w389, index=13) -> (element=w411:T1)
                  n184 = Index Array(array=w389, index=14) -> (element=w395:T1)
                  n185 = Index Array(array=w389, index=15) -> (element=w400:T1)
                  n186 = Index Array(array=w389, index=0) -> (element=w526:T1)
                  n187 = Index Array(array=w389, index=1) -> (element=w521:T1)
                  n188 = Index Array(array=w389, index=2) -> (element=w503:T1)
                  n189 = Index Array(array=w389, index=3) -> (element=w508:T1)
                  n190 = Index Array(array=w389, index=4) -> (element=w490:T1)
                  n191 = Index Array(array=w389, index=5) -> (element=w485:T1)
                  n192 = Index Array(array=w389, index=6) -> (element=w467:T1)
                  n193 = Index Array(array=w389, index=7) -> (element=w472:T1)
                  n194 = Index Array(array=w389, index=8) -> (element=w452:T1)
                  n195 = Index Array(array=w389, index=9) -> (element=w447:T1)
                  n196 = Index Array(array=w389, index=10) -> (element=w430:T1)
                  n197 = Index Array(array=w389, index=11) -> (element=w435:T1)
                  n198 = disable-structure shown="FPGA_TARGET_CLASS==USRP_X410||FPGA_TARGET_CLASS==USRP_X410__EMBEDDED____UNSUPPORTED" {
                    disable-tunnel: [refnum<k21> "RF 0/Tx/I" ("tx regs.i out resource") refnum<k21> "Daughterboard 0\\RF 0.Tx.I0" ("FPGA I/O")] -> w388
                    disable-tunnel: [refnum<k21> "RF 0/Tx/Q" ("tx regs.i out resource") refnum<k21> "Daughterboard 0\\RF 0.Tx.Q0" ("FPGA I/O")] -> w387
                    frame condition #0 {
                    }
                    frame condition #1 (active) {
                    }
                  }
                  n199 = disable-structure shown="FPGA_TARGET_CLASS==USRP_X410||FPGA_TARGET_CLASS==USRP_X410__EMBEDDED____UNSUPPORTED" {
                    disable-tunnel: [refnum<k21> "RF 0/Tx/I" ("tx regs.i out resource") refnum<k21> "Daughterboard 0\\RF 0.Tx.I1" ("FPGA I/O")] -> w386
                    disable-tunnel: [refnum<k21> "RF 0/Tx/Q" ("tx regs.i out resource") refnum<k21> "Daughterboard 0\\RF 0.Tx.Q1" ("FPGA I/O")] -> w385
                    frame condition #0 {
                    }
                    frame condition #1 (active) {
                    }
                  }
                  n200 = disable-structure shown="FPGA_TARGET_CLASS==USRP_X410||FPGA_TARGET_CLASS==USRP_X410__EMBEDDED____UNSUPPORTED" {
                    disable-tunnel: [refnum<k21> "RF 0/Tx/I" ("tx regs.i out resource") refnum<k21> "Daughterboard 0\\RF 0.Tx.I2" ("FPGA I/O")] -> w384
                    disable-tunnel: [refnum<k21> "RF 0/Tx/Q" ("tx regs.i out resource") refnum<k21> "Daughterboard 0\\RF 0.Tx.Q2" ("FPGA I/O")] -> w383
                    frame condition #0 {
                    }
                    frame condition #1 (active) {
                    }
                  }
                  n201 = disable-structure shown="FPGA_TARGET_CLASS==USRP_X410||FPGA_TARGET_CLASS==USRP_X410__EMBEDDED____UNSUPPORTED" {
                    disable-tunnel: [refnum<k21> "RF 0/Tx/I" ("tx regs.i out resource") refnum<k21> "Daughterboard 0\\RF 0.Tx.I3" ("FPGA I/O")] -> w382
                    disable-tunnel: [refnum<k21> "RF 0/Tx/Q" ("tx regs.i out resource") refnum<k21> "Daughterboard 0\\RF 0.Tx.Q3" ("FPGA I/O")] -> w381
                    frame condition #0 {
                    }
                    frame condition #1 (active) {
                    }
                  }
                  n202 = disable-structure shown="FPGA_TARGET_CLASS==USRP_X410||FPGA_TARGET_CLASS==USRP_X410__EMBEDDED____UNSUPPORTED" {
                    disable-tunnel: [refnum<k21> "RF 0/Tx/I" ("tx regs.i out resource") refnum<k21> "Daughterboard 0\\RF 1.Tx.I0" ("FPGA I/O")] -> w380
                    disable-tunnel: [refnum<k21> "RF 0/Tx/Q" ("tx regs.i out resource") refnum<k21> "Daughterboard 0\\RF 1.Tx.Q0" ("FPGA I/O")] -> w379
                    frame condition #0 {
                    }
                    frame condition #1 (active) {
                    }
                  }
                  n203 = disable-structure shown="FPGA_TARGET_CLASS==USRP_X410||FPGA_TARGET_CLASS==USRP_X410__EMBEDDED____UNSUPPORTED" {
                    disable-tunnel: [refnum<k21> "RF 0/Tx/I" ("tx regs.i out resource") refnum<k21> "Daughterboard 0\\RF 1.Tx.I1" ("FPGA I/O")] -> w378
                    disable-tunnel: [refnum<k21> "RF 0/Tx/Q" ("tx regs.i out resource") refnum<k21> "Daughterboard 0\\RF 1.Tx.Q1" ("FPGA I/O")] -> w377
                    frame condition #0 {
                    }
                    frame condition #1 (active) {
                    }
                  }
                  n204 = disable-structure shown="FPGA_TARGET_CLASS==USRP_X410||FPGA_TARGET_CLASS==USRP_X410__EMBEDDED____UNSUPPORTED" {
                    disable-tunnel: [refnum<k21> "RF 0/Tx/I" ("tx regs.i out resource") refnum<k21> "Daughterboard 0\\RF 1.Tx.I2" ("FPGA I/O")] -> w376
                    disable-tunnel: [refnum<k21> "RF 0/Tx/Q" ("tx regs.i out resource") refnum<k21> "Daughterboard 0\\RF 1.Tx.Q2" ("FPGA I/O")] -> w375
                    frame condition #0 {
                    }
                    frame condition #1 (active) {
                    }
                  }
                  n205 = disable-structure shown="FPGA_TARGET_CLASS==USRP_X410||FPGA_TARGET_CLASS==USRP_X410__EMBEDDED____UNSUPPORTED" {
                    disable-tunnel: [refnum<k21> "RF 0/Tx/I" ("tx regs.i out resource") refnum<k21> "Daughterboard 1\\RF 0.Tx.I0" ("FPGA I/O")] -> w372
                    disable-tunnel: [refnum<k21> "RF 0/Tx/Q" ("tx regs.i out resource") refnum<k21> "Daughterboard 1\\RF 0.Tx.Q0" ("FPGA I/O")] -> w371
                    frame condition #0 {
                    }
                    frame condition #1 (active) {
                    }
                  }
                  n206 = disable-structure shown="FPGA_TARGET_CLASS==USRP_X410||FPGA_TARGET_CLASS==USRP_X410__EMBEDDED____UNSUPPORTED" {
                    disable-tunnel: [refnum<k21> "RF 0/Tx/I" ("tx regs.i out resource") refnum<k21> "Daughterboard 0\\RF 1.Tx.I3" ("FPGA I/O")] -> w374
                    disable-tunnel: [refnum<k21> "RF 0/Tx/Q" ("tx regs.i out resource") refnum<k21> "Daughterboard 0\\RF 1.Tx.Q3" ("FPGA I/O")] -> w373
                    frame condition #0 {
                    }
                    frame condition #1 (active) {
                    }
                  }
                  n207 = disable-structure shown="FPGA_TARGET_CLASS==USRP_X410||FPGA_TARGET_CLASS==USRP_X410__EMBEDDED____UNSUPPORTED" {
                    disable-tunnel: [refnum<k21> "RF 0/Tx/I" ("tx regs.i out resource") refnum<k21> "Daughterboard 1\\RF 0.Tx.I1" ("FPGA I/O")] -> w370
                    disable-tunnel: [refnum<k21> "RF 0/Tx/Q" ("tx regs.i out resource") refnum<k21> "Daughterboard 1\\RF 0.Tx.Q1" ("FPGA I/O")] -> w369
                    frame condition #0 {
                    }
                    frame condition #1 (active) {
                    }
                  }
                  n208 = disable-structure shown="FPGA_TARGET_CLASS==USRP_X410||FPGA_TARGET_CLASS==USRP_X410__EMBEDDED____UNSUPPORTED" {
                    disable-tunnel: [refnum<k21> "RF 0/Tx/I" ("tx regs.i out resource") refnum<k21> "Daughterboard 1\\RF 0.Tx.I2" ("FPGA I/O")] -> w353
                    disable-tunnel: [refnum<k21> "RF 0/Tx/Q" ("tx regs.i out resource") refnum<k21> "Daughterboard 1\\RF 0.Tx.Q2" ("FPGA I/O")] -> w352
                    frame condition #0 {
                    }
                    frame condition #1 (active) {
                    }
                  }
                  n209 = disable-structure shown="FPGA_TARGET_CLASS==USRP_X410||FPGA_TARGET_CLASS==USRP_X410__EMBEDDED____UNSUPPORTED" {
                    disable-tunnel: [refnum<k21> "RF 0/Tx/I" ("tx regs.i out resource") refnum<k21> "Daughterboard 1\\RF 1.Tx.I0" ("FPGA I/O")] -> w357
                    disable-tunnel: [refnum<k21> "RF 0/Tx/Q" ("tx regs.i out resource") refnum<k21> "Daughterboard 1\\RF 1.Tx.Q0" ("FPGA I/O")] -> w356
                    frame condition #0 {
                    }
                    frame condition #1 (active) {
                    }
                  }
                  n210 = disable-structure shown="FPGA_TARGET_CLASS==USRP_X410||FPGA_TARGET_CLASS==USRP_X410__EMBEDDED____UNSUPPORTED" {
                    disable-tunnel: [refnum<k21> "RF 0/Tx/Q" ("tx regs.i out resource") refnum<k21> "Daughterboard 1\\RF 0.Tx.Q3" ("FPGA I/O")] -> w350
                    disable-tunnel: [refnum<k21> "RF 0/Tx/I" ("tx regs.i out resource") refnum<k21> "Daughterboard 1\\RF 0.Tx.I3" ("FPGA I/O")] -> w351
                    frame condition #0 {
                    }
                    frame condition #1 (active) {
                    }
                  }
                  n211 = disable-structure shown="FPGA_TARGET_CLASS==USRP_X410||FPGA_TARGET_CLASS==USRP_X410__EMBEDDED____UNSUPPORTED" {
                    disable-tunnel: [refnum<k21> "RF 0/Tx/I" ("tx regs.i out resource") refnum<k21> "Daughterboard 1\\RF 1.Tx.I1" ("FPGA I/O")] -> w359
                    disable-tunnel: [refnum<k21> "RF 0/Tx/Q" ("tx regs.i out resource") refnum<k21> "Daughterboard 1\\RF 1.Tx.Q1" ("FPGA I/O")] -> w358
                    frame condition #0 {
                    }
                    frame condition #1 (active) {
                    }
                  }
                  n212 = disable-structure shown="FPGA_TARGET_CLASS==USRP_X410||FPGA_TARGET_CLASS==USRP_X410__EMBEDDED____UNSUPPORTED" {
                    disable-tunnel: [refnum<k21> "RF 0/Tx/I" ("tx regs.i out resource") refnum<k21> "Daughterboard 1\\RF 1.Tx.I2" ("FPGA I/O")] -> w363
                    disable-tunnel: [refnum<k21> "RF 0/Tx/Q" ("tx regs.i out resource") refnum<k21> "Daughterboard 1\\RF 1.Tx.Q2" ("FPGA I/O")] -> w362
                    frame condition #0 {
                    }
                    frame condition #1 (active) {
                    }
                  }
                  n213 = disable-structure shown="FPGA_TARGET_CLASS==USRP_X410||FPGA_TARGET_CLASS==USRP_X410__EMBEDDED____UNSUPPORTED" {
                    disable-tunnel: [refnum<k21> "RF 0/Tx/I" ("tx regs.i out resource") refnum<k21> "Daughterboard 1\\RF 1.Tx.I3" ("FPGA I/O")] -> w366
                    disable-tunnel: [refnum<k21> "RF 0/Tx/Q" ("tx regs.i out resource") refnum<k21> "Daughterboard 1\\RF 1.Tx.Q3" ("FPGA I/O")] -> w367
                    frame condition #0 {
                    }
                    frame condition #1 (active) {
                    }
                  }
                  n214 = Build Array(w416) -> (w414:T1[])
                  n215 = Build Array(w411) -> (w413:T1[])
                  n216 = Build Array(w395) -> (w397:T1[])
                  n217 = Build Array(w400) -> (w398:T1[])
                  n218 = Build Array(w526) -> (w524:T1[])
                  n219 = Build Array(w521) -> (w523:T1[])
                  n220 = Build Array(w503) -> (w505:T1[])
                  n221 = Build Array(w508) -> (w506:T1[])
                  n222 = Build Array(w490) -> (w488:T1[])
                  n223 = Build Array(w485) -> (w487:T1[])
                  n224 = Build Array(w467) -> (w469:T1[])
                  n225 = Build Array(w472) -> (w470:T1[])
                  n226 = Build Array(w452) -> (w450:T1[])
                  n227 = Build Array(w447) -> (w449:T1[])
                  n228 = Build Array(w430) -> (w432:T1[])
                  n229 = Build Array(w435) -> (w433:T1[])
                  n230 = call "IQ Data to IO Node - S16.1 - N spc.vi"("data in"=w414) -> ("I out"=w424:fxp<+/-,16,1>[], "Q out"=w423:fxp<+/-,16,1>[])  [unwired: 12 in, 1 out]
                  n231 = call "IQ Data to IO Node - S16.1 - N spc.vi"("data in"=w413) -> ("I out"=w406:fxp<+/-,16,1>[], "Q out"=w407:fxp<+/-,16,1>[])  [unwired: 12 in, 1 out]
                  n232 = call "IQ Data to IO Node - S16.1 - N spc.vi"("data in"=w397) -> ("I out"=w390:fxp<+/-,16,1>[], "Q out"=w391:fxp<+/-,16,1>[])  [unwired: 12 in, 1 out]
                  n233 = call "IQ Data to IO Node - S16.1 - N spc.vi"("data in"=w398) -> ("I out"=w405:fxp<+/-,16,1>[], "Q out"=w404:fxp<+/-,16,1>[])  [unwired: 12 in, 1 out]
                  n234 = call "IQ Data to IO Node - S16.1 - N spc.vi"("data in"=w524) -> ("I out"=w534:fxp<+/-,16,1>[], "Q out"=w533:fxp<+/-,16,1>[])  [unwired: 12 in, 1 out]
                  n235 = call "IQ Data to IO Node - S16.1 - N spc.vi"("data in"=w523) -> ("I out"=w515:fxp<+/-,16,1>[], "Q out"=w516:fxp<+/-,16,1>[])  [unwired: 12 in, 1 out]
                  n236 = call "IQ Data to IO Node - S16.1 - N spc.vi"("data in"=w505) -> ("I out"=w497:fxp<+/-,16,1>[], "Q out"=w498:fxp<+/-,16,1>[])  [unwired: 12 in, 1 out]
                  n237 = call "IQ Data to IO Node - S16.1 - N spc.vi"("data in"=w506) -> ("I out"=w514:fxp<+/-,16,1>[], "Q out"=w513:fxp<+/-,16,1>[])  [unwired: 12 in, 1 out]
                  n238 = call "IQ Data to IO Node - S16.1 - N spc.vi"("data in"=w488) -> ("I out"=w496:fxp<+/-,16,1>[], "Q out"=w495:fxp<+/-,16,1>[])  [unwired: 12 in, 1 out]
                  n239 = call "IQ Data to IO Node - S16.1 - N spc.vi"("data in"=w487) -> ("I out"=w479:fxp<+/-,16,1>[], "Q out"=w480:fxp<+/-,16,1>[])  [unwired: 12 in, 1 out]
                  n240 = call "IQ Data to IO Node - S16.1 - N spc.vi"("data in"=w469) -> ("I out"=w461:fxp<+/-,16,1>[], "Q out"=w462:fxp<+/-,16,1>[])  [unwired: 12 in, 1 out]
                  n241 = call "IQ Data to IO Node - S16.1 - N spc.vi"("data in"=w470) -> ("I out"=w478:fxp<+/-,16,1>[], "Q out"=w477:fxp<+/-,16,1>[])  [unwired: 12 in, 1 out]
                  n242 = call "IQ Data to IO Node - S16.1 - N spc.vi"("data in"=w450) -> ("I out"=w460:fxp<+/-,16,1>[], "Q out"=w459:fxp<+/-,16,1>[])  [unwired: 12 in, 1 out]
                  n243 = call "IQ Data to IO Node - S16.1 - N spc.vi"("data in"=w449) -> ("I out"=w441:fxp<+/-,16,1>[], "Q out"=w442:fxp<+/-,16,1>[])  [unwired: 12 in, 1 out]
                  n244 = call "IQ Data to IO Node - S16.1 - N spc.vi"("data in"=w432) -> ("I out"=w425:fxp<+/-,16,1>[], "Q out"=w426:fxp<+/-,16,1>[])  [unwired: 12 in, 1 out]
                  n245 = call "IQ Data to IO Node - S16.1 - N spc.vi"("data in"=w433) -> ("I out"=w440:fxp<+/-,16,1>[], "Q out"=w439:fxp<+/-,16,1>[])  [unwired: 12 in, 1 out]
                  n246 = Index Array(array=w424, index=w419) -> (element=w422:fxp<+/-,16,1>)
                  n247 = Index Array(array=w423, index=w419) -> (element=w420:fxp<+/-,16,1>)
                  n248 = Index Array(array=w406, index=w410) -> (element=w408:fxp<+/-,16,1>)
                  n249 = Index Array(array=w407, index=w410) -> (element=w409:fxp<+/-,16,1>)
                  n250 = Index Array(array=w390, index=w394) -> (element=w392:fxp<+/-,16,1>)
                  n251 = Index Array(array=w391, index=w394) -> (element=w393:fxp<+/-,16,1>)
                  n252 = Index Array(array=w405, index=w401) -> (element=w403:fxp<+/-,16,1>)
                  n253 = Index Array(array=w404, index=w401) -> (element=w402:fxp<+/-,16,1>)
                  n254 = Index Array(array=w534, index=w529) -> (element=w532:fxp<+/-,16,1>)
                  n255 = Index Array(array=w533, index=w529) -> (element=w530:fxp<+/-,16,1>)
                  n256 = Index Array(array=w515, index=w520) -> (element=w517:fxp<+/-,16,1>)
                  n257 = Index Array(array=w516, index=w520) -> (element=w519:fxp<+/-,16,1>)
                  n258 = Index Array(array=w497, index=w501) -> (element=w499:fxp<+/-,16,1>)
                  n259 = Index Array(array=w498, index=w501) -> (element=w500:fxp<+/-,16,1>)
                  n260 = Index Array(array=w514, index=w510) -> (element=w512:fxp<+/-,16,1>)
                  n261 = Index Array(array=w513, index=w510) -> (element=w511:fxp<+/-,16,1>)
                  n262 = Index Array(array=w496, index=w492) -> (element=w494:fxp<+/-,16,1>)
                  n263 = Index Array(array=w495, index=w492) -> (element=w493:fxp<+/-,16,1>)
                  n264 = Index Array(array=w479, index=w483) -> (element=w481:fxp<+/-,16,1>)
                  n265 = Index Array(array=w480, index=w483) -> (element=w482:fxp<+/-,16,1>)
                  n266 = Index Array(array=w461, index=w465) -> (element=w463:fxp<+/-,16,1>)
                  n267 = Index Array(array=w462, index=w465) -> (element=w464:fxp<+/-,16,1>)
                  n268 = Index Array(array=w478, index=w474) -> (element=w476:fxp<+/-,16,1>)
                  n269 = Index Array(array=w477, index=w474) -> (element=w475:fxp<+/-,16,1>)
                  n270 = Index Array(array=w460, index=w455) -> (element=w458:fxp<+/-,16,1>)
                  n271 = Index Array(array=w459, index=w455) -> (element=w456:fxp<+/-,16,1>)
                  n272 = Index Array(array=w441, index=w446) -> (element=w443:fxp<+/-,16,1>)
                  n273 = Index Array(array=w442, index=w446) -> (element=w445:fxp<+/-,16,1>)
                  n274 = Index Array(array=w425, index=w429) -> (element=w427:fxp<+/-,16,1>)
                  n275 = Index Array(array=w440, index=w436) -> (element=w438:fxp<+/-,16,1>)
                  n276 = Index Array(array=w439, index=w436) -> (element=w437:fxp<+/-,16,1>)
                  n277 = Index Array(array=w426, index=w429) -> (element=w428:fxp<+/-,16,1>)
                  n278 = Fixed-Point to Integer Cast(1:w532) -> (0:w531:i16)
                  n279 = Fixed-Point to Integer Cast(1:w530) -> (0:w528:i16)
                  n280 = Fixed-Point to Integer Cast(1:w517) -> (0:w518:i16)
                  n281 = Fixed-Point to Integer Cast(1:w519) -> (0:w341:i16)
                  n282 = Fixed-Point to Integer Cast(1:w499) -> (0:w340:i16)
                  n283 = Fixed-Point to Integer Cast(1:w500) -> (0:w502:i16)
                  n284 = Fixed-Point to Integer Cast(1:w512) -> (0:w342:i16)
                  n285 = Fixed-Point to Integer Cast(1:w511) -> (0:w509:i16)
                  n286 = Fixed-Point to Integer Cast(1:w494) -> (0:w344:i16)
                  n287 = Fixed-Point to Integer Cast(1:w493) -> (0:w343:i16)
                  n288 = Fixed-Point to Integer Cast(1:w481) -> (0:w339:i16)
                  n289 = Fixed-Point to Integer Cast(1:w482) -> (0:w484:i16)
                  n290 = Fixed-Point to Integer Cast(1:w463) -> (0:w338:i16)
                  n291 = Fixed-Point to Integer Cast(1:w464) -> (0:w466:i16)
                  n292 = Fixed-Point to Integer Cast(1:w476) -> (0:w345:i16)
                  n293 = Fixed-Point to Integer Cast(1:w475) -> (0:w473:i16)
                  n294 = Fixed-Point to Integer Cast(1:w458) -> (0:w457:i16)
                  n295 = Fixed-Point to Integer Cast(1:w456) -> (0:w454:i16)
                  n296 = Fixed-Point to Integer Cast(1:w443) -> (0:w444:i16)
                  n297 = Fixed-Point to Integer Cast(1:w445) -> (0:w368:i16)
                  n298 = Fixed-Point to Integer Cast(1:w427) -> (0:w346:i16)
                  n299 = Fixed-Point to Integer Cast(1:w428) -> (0:w347:i16)
                  n300 = Fixed-Point to Integer Cast(1:w438) -> (0:w349:i16)
                  n301 = Fixed-Point to Integer Cast(1:w437) -> (0:w348:i16)
                  n302 = Fixed-Point to Integer Cast(1:w422) -> (0:w421:i16)
                  n303 = Fixed-Point to Integer Cast(1:w420) -> (0:w418:i16)
                  n304 = Fixed-Point to Integer Cast(1:w408) -> (0:w355:i16)
                  n305 = Fixed-Point to Integer Cast(1:w409) -> (0:w354:i16)
                  n306 = Fixed-Point to Integer Cast(1:w392) -> (0:w361:i16)
                  n307 = Fixed-Point to Integer Cast(1:w393) -> (0:w360:i16)
                  n308 = Fixed-Point to Integer Cast(1:w403) -> (0:w365:i16)
                  n309 = Fixed-Point to Integer Cast(1:w402) -> (0:w364:i16)
                  n310 = xnode "FPGA I/O Node"("I/O Item"=w421, "FPGA I/O In"=w357, "I/O Item"=w418, "FPGA I/O In"=w356, "Daughterboard 1\\RF 1.Tx.Data Valid"=TRUE ("Daughterboard 1\\s1TxDbaCh0DataValid")) -> ()  [unwired: 1 in, 3 out]
                  n311 = xnode "FPGA I/O Node"("I/O Item"=w355, "FPGA I/O In"=w359, "I/O Item"=w354, "FPGA I/O In"=w358) -> ()  [unwired: 2 out]
                  n312 = xnode "FPGA I/O Node"("I/O Item"=w361, "FPGA I/O In"=w363, "I/O Item"=w360, "FPGA I/O In"=w362) -> ()  [unwired: 2 out]
                  n313 = xnode "FPGA I/O Node"("I/O Item"=w365, "FPGA I/O In"=w366, "I/O Item"=w364, "FPGA I/O In"=w367) -> ()  [unwired: 2 out]
                  n314 = xnode "FPGA I/O Node"("I/O Item"=w531, "FPGA I/O In"=w388, "I/O Item"=w528, "FPGA I/O In"=w387, "Daughterboard 0\\RF 0.Tx.Data Valid"=TRUE ("Daughterboard 1\\s1TxDbaCh0DataValid")) -> ()  [unwired: 1 in, 3 out]
                  n315 = xnode "FPGA I/O Node"("I/O Item"=w518, "FPGA I/O In"=w386, "I/O Item"=w341, "FPGA I/O In"=w385) -> ()  [unwired: 2 out]
                  n316 = xnode "FPGA I/O Node"("I/O Item"=w340, "FPGA I/O In"=w384, "I/O Item"=w502, "FPGA I/O In"=w383) -> ()  [unwired: 2 out]
                  n317 = xnode "FPGA I/O Node"("I/O Item"=w342, "FPGA I/O In"=w382, "I/O Item"=w509, "FPGA I/O In"=w381) -> ()  [unwired: 2 out]
                  n318 = xnode "FPGA I/O Node"("I/O Item"=w344, "FPGA I/O In"=w380, "I/O Item"=w343, "FPGA I/O In"=w379, "Daughterboard 0\\RF 1.Tx.Data Valid"=TRUE ("Daughterboard 1\\s1TxDbaCh0DataValid")) -> ()  [unwired: 1 in, 3 out]
                  n319 = xnode "FPGA I/O Node"("I/O Item"=w339, "FPGA I/O In"=w378, "I/O Item"=w484, "FPGA I/O In"=w377) -> ()  [unwired: 2 out]
                  n320 = xnode "FPGA I/O Node"("I/O Item"=w338, "FPGA I/O In"=w376, "I/O Item"=w466, "FPGA I/O In"=w375) -> ()  [unwired: 2 out]
                  n321 = xnode "FPGA I/O Node"("I/O Item"=w345, "FPGA I/O In"=w374, "I/O Item"=w473, "FPGA I/O In"=w373) -> ()  [unwired: 2 out]
                  n322 = xnode "FPGA I/O Node"("I/O Item"=w457, "FPGA I/O In"=w372, "I/O Item"=w454, "FPGA I/O In"=w371, "Daughterboard 1\\RF 0.Tx.Data Valid"=TRUE ("Daughterboard 1\\s1TxDbaCh0DataValid")) -> ()  [unwired: 1 in, 3 out]
                  n323 = xnode "FPGA I/O Node"("I/O Item"=w444, "FPGA I/O In"=w370, "I/O Item"=w368, "FPGA I/O In"=w369) -> ()  [unwired: 2 out]
                  n324 = xnode "FPGA I/O Node"("I/O Item"=w346, "FPGA I/O In"=w353, "I/O Item"=w347, "FPGA I/O In"=w352) -> ()  [unwired: 2 out]
                  n325 = xnode "FPGA I/O Node"("I/O Item"=w349, "FPGA I/O In"=w351, "I/O Item"=w348, "FPGA I/O In"=w350) -> ()  [unwired: 2 out]
                }
              }
            }
            frame condition #1 {
              n326 = Unbundle By Name(w612) -> ("Loopback FIFO"=w621:refnum<k21>)
              n327 = Array Size(array=w611) -> (size(s)=w620:i32)
              n328 = Initialize Array(T1 {"I"=0.0, "Q"=0.0, "overflow"=FALSE} ("data"), w620) -> (w618:T1[])
              n329 = feedback #1(w618) -> (w616:T1[])
              n330 = feedback-in #1(w611) -> ()
              n331 = Index Array(array=w616) -> (element #1=w615:T1, element #2=w614:T1, element #3=w610:T1, element #4=w609:T1)  [unwired: 4 in]
              n332 = call <instrlib>:"IQ to U32 - 1 spc - S18.1.vi"("IQ data"=w615) -> ("U32 data"=w613:u32)  [unwired: 13 in, 1 out]
              n333 = call <instrlib>:"IQ to U32 - 1 spc - S18.1.vi"("IQ data"=w614) -> ("U32 data"=w605:u32)  [unwired: 13 in, 1 out]
              n334 = call <instrlib>:"IQ to U32 - 1 spc - S18.1.vi"("IQ data"=w610) -> ("U32 data"=w604:u32)  [unwired: 13 in, 1 out]
              n335 = call <instrlib>:"IQ to U32 - 1 spc - S18.1.vi"("IQ data"=w609) -> ("U32 data"=w603:u32)  [unwired: 13 in, 1 out]
              n336 = To Unsigned Word Integer(number=w613) -> (unsigned 16bit integer=w606:u16)
              n337 = To Unsigned Word Integer(number=w605) -> (unsigned 16bit integer=w602:u16)
              n338 = To Unsigned Word Integer(number=w604) -> (unsigned 16bit integer=w601:u16)
              n339 = To Unsigned Word Integer(number=w603) -> (unsigned 16bit integer=w600:u16)
              n340 = Join Numbers(hi=w606, lo=w602) -> ((hi.lo)=w608:u32)
              n341 = Join Numbers(hi=w601, lo=w600) -> ((hi.lo)=w599:u32)
              n342 = Join Numbers(hi=w608, lo=w599) -> ((hi.lo)=w607:u64)
              n343 = xnode ("FIFO Write")("Element"=w607, "Timeout"=0, "FIFO In"=w621) -> ()  [unwired: 2 out]
            }
          }
        }
      }
    }
    frame condition #2 {
    }
  }
